vi "HTTPS Server Test.vi"() -> ()   [LabVIEW 2013]
uses:
  NI OpenSSL Socket/SSL_Lib/SSL-Lib/Library Paths.ctl
  NI OpenSSL Socket/SSL_Lib/SSL/SSL_Mode.ctl
  NI OpenSSL Socket/SSL_Lib/SSL-Lib/SSL-Lib.lvclass
  NI OpenSSL Socket/SSL_Lib/SSL-Context/SSL-Context.lvclass
  NI OpenSSL Socket/SSL_Lib/BIO/BIO.lvclass
  NI OpenSSL Socket/SSL_Lib/SSL/SSL.lvclass
panel:
  out "listener":i32
  out "accept":i32
  in  "String write":string="Hello!"
  out "String read":string
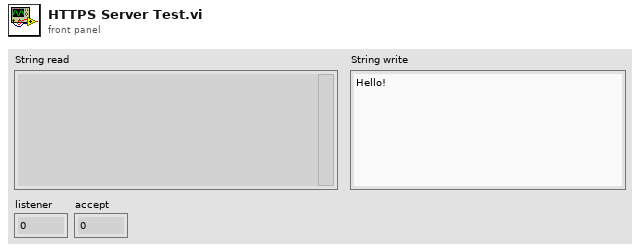
[diagram p1: front panel]
types:
  T1 = typedef "OpenSSL Socket.lvlib/SSL.lvclass/SSL_Mode.ctl" = i32
  T2 = typedef "OpenSSL Socket.lvlib/SSL-Lib.lvclass/Library Paths.ctl" = cluster{"SSL Library Path":path, "Crypto Library Path":path}
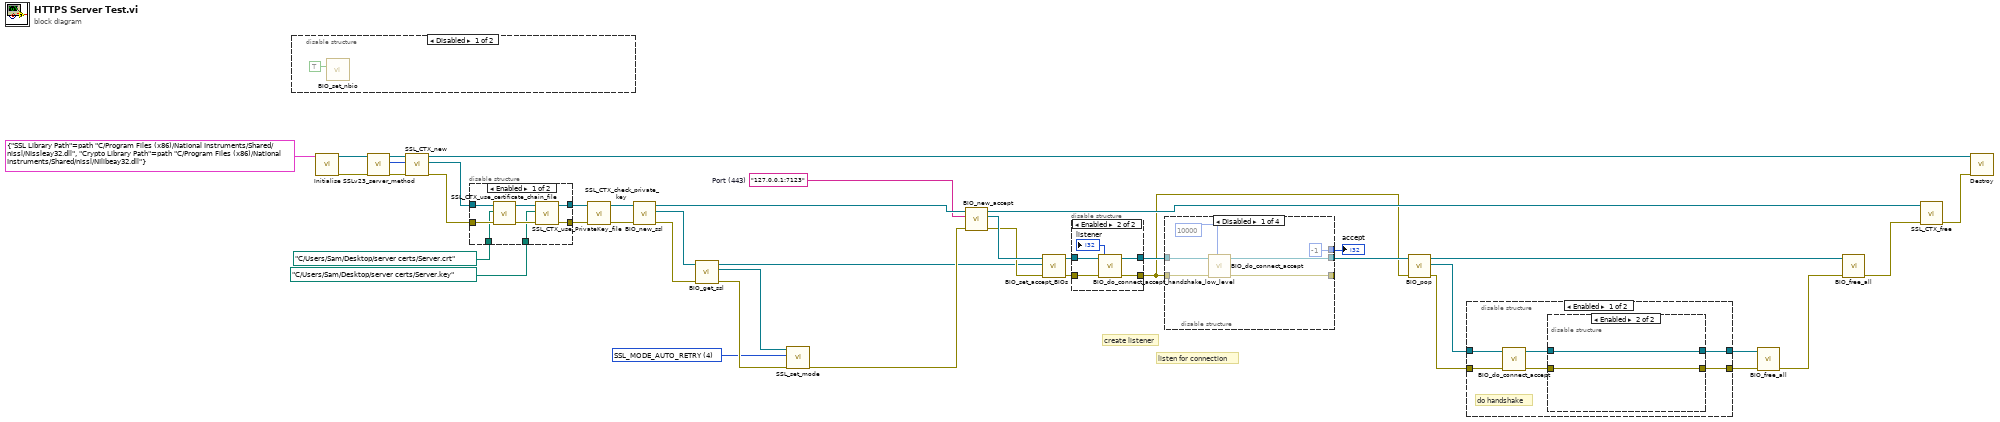
[diagram p0: block diagram]
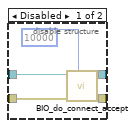
[diagram p2: hidden frame]
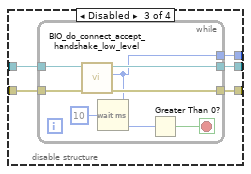
[diagram p4: hidden frame]
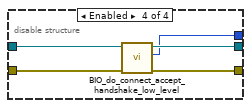
[diagram p5: hidden frame]
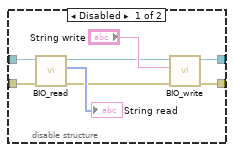
[diagram p6: hidden frame]
diagram:
  w15 = "127.0.0.1:7123"  # Port (443)
  w22 = T1 4 items=["None"=0, "SSL_MODE_ENABLE_PARTIAL_WRITE"=1, "SSL_MODE_ACCEPT_MOVING_WRITE_BUFFER"=2, "SSL_MODE_AUTO_RETRY"=4, "SSL_MODE_RELEASE_BUFFERS"=16, "SSL_MODE_SEND_FALLBACK_SCSV"=128] ("Mode")
  # "listen for connection"
  # "create listener"
  n1 = disable-structure shown="Disabled" {
    frame Disabled {
      n2 = call "BIO_set_nbio.vi"("Non-Blocking?"=TRUE) -> ()  [unwired: 9 in, 2 out]
    }
    frame Enabled {
    }
  }
  n3 = call "Initialise.vi"("Library Paths"=T2 {"SSL Library Path"=path "C:/Program Files (x86)/National Instruments/Shared/nissl/NIssleay32.dll", "Crypto Library Path"=path "C:/Program Files (x86)/National Instruments/Shared/nissl/NIlibeay32.dll"}) -> ("error out"=w37:errorcluster, "SSL-Lib out"=w41:refnum<class "SSL-Lib.lvclass">)  [unwired: 9 in]
  n4 = call "SSLv23_server_method.vi"("error in (no error)"=w37, "SSL-Lib in"=w41) -> ("error out"=w35:errorcluster, "*SSL_Method"=w40:u64, "SSL-Lib out"=w39:refnum<class "SSL-Lib.lvclass">)  [unwired: 7 in]
  n5 = call "SSL_CTX_new.vi"("error in (no error)"=w35, "*SSL_Method"=w40, "SSL-Lib in"=w39) -> ("error out"=w34:errorcluster, "SSL-Context out"=w33:refnum<class "SSL-Context.lvclass">, "SSL-Lib out"=w4:refnum<class "SSL-Lib.lvclass">)  [unwired: 6 in]
  n6 = disable-structure shown="Enabled" {
    disable-tunnel: w34 -> [w48 w51]
    disable-tunnel: w33 -> [w47 w52]
    disable-tunnel: [w46 w51] -> w32
    disable-tunnel: [w45 w52] -> w31
    disable-tunnel: path "C:/Users/Sam/Desktop/server certs/Server.crt" -> [w44 _]
    disable-tunnel: path "C:/Users/Sam/Desktop/server certs/Server.key" -> [w43 _]
    frame Enabled {
      n7 = call "SSL_CTX_use_certificate_chain_file.vi"("error in (no error)"=w48, "Certificate Chain File"=w44, "SSL-Context in"=w47) -> ("error out"=w50:errorcluster, "SSL-Context out"=w49:refnum<class "SSL-Context.lvclass">)  [unwired: 7 in]
      n8 = call "SSL_CTX_use_PrivateKey_file.vi"("error in (no error)"=w50, "PrivateKey File"=w43, "SSL-Context in"=w49) -> ("error out"=w46:errorcluster, "SSL-Context out"=w45:refnum<class "SSL-Context.lvclass">)  [unwired: 7 in]
    }
    frame Disabled {
    }
  }
  n9 = call "SSL_CTX_check_private_key.vi"("error in (no error)"=w32, "SSL-Context in"=w31) -> ("error out"=w30:errorcluster, "SSL-Context out"=w29:refnum<class "SSL-Context.lvclass">)  [unwired: 8 in]
  n10 = call "BIO_new_ssl.vi"("error in (no error)"=w30, "SSL-Context in"=w29) -> ("error out"=w25:errorcluster, "SSL BIO out"=w26:refnum<class "BIO.lvclass">, "SSL-Context out"=w19:refnum<class "SSL-Context.lvclass">)  [unwired: 7 in]
  n11 = call "BIO_get_ssl.vi"("error in (no error)"=w25, "BIO in"=w26) -> ("error out"=w23:errorcluster, "SSL out"=w24:refnum<class "SSL.lvclass">, "BIO out"=w2:refnum<class "BIO.lvclass">)  [unwired: 7 in]
  n12 = call "SSL_set_mode.vi"("error in (no error)"=w23, "Mode"=w22, "SSL in"=w24) -> ("error out"=w3:errorcluster)  [unwired: 7 in, 1 out]
  n13 = call "BIO_new_accept.vi"("error in (no error)"=w3, "Port (443)"=w15, "SSL-Context in"=w19) -> ("error out"=w16:errorcluster, "Accept BIO out"=w17:refnum<class "BIO.lvclass">, "SSL-Context out"=w18:refnum<class "SSL-Context.lvclass">)  [unwired: 6 in]
  n14 = call "BIO_set_accept_BIOs.vi"("error in (no error)"=w16, "SSL BIO"=w2, "Accept BIO in"=w17) -> ("error out"=w13:errorcluster, "Accept BIO out"=w14:refnum<class "BIO.lvclass">)  [unwired: 7 in]
  n15 = disable-structure shown="Enabled" {
    disable-tunnel: w14 -> [w56 w62]
    disable-tunnel: w13 -> [w55 w61]
    disable-tunnel: [w54 w59] -> w12
    disable-tunnel: [w53 w60] -> w5
    frame Disabled {
      n16 = call "BIO_do_connect_accept.vi"(7:u32 10000 ("Timeout (10000ms)"), "error in (no error)"=w55, "BIO in"=w56) -> ("error out"=w53:errorcluster, "BIO out"=w54:refnum<class "BIO.lvclass">)  [unwired: 7 in]
    }
    frame Enabled {
      n17 = call "BIO_do_connect_accept_handshake_low_level.vi"("error in (no error)"=w61, "BIO in"=w62) -> ("error out"=w60:errorcluster, "return type"=→"listener":i32, "BIO out"=w59:refnum<class "BIO.lvclass">)  [unwired: 7 in]
    }
  }
  n18 = disable-structure shown="Disabled" {
    disable-tunnel: w12 -> [w67 w70 w75 w87]
    disable-tunnel: w5 -> [w66 w69 w74 w86]
    disable-tunnel: [w65 w70 w73 w85] -> w10
    disable-tunnel: [w64 w69 w72 w84] -> _
    disable-tunnel: [-1 ("return type") _ w71 w83] -> w1
    frame Disabled {
      n19 = call "BIO_do_connect_accept.vi"(7:u32 10000 ("Timeout (10000ms)"), "error in (no error)"=w66, "BIO in"=w67) -> ("error out"=w64:errorcluster, "BIO out"=w65:refnum<class "BIO.lvclass">)  [unwired: 7 in]
    }
    frame Disabled {
    }
    frame Disabled {
      n20 = while {
        tunnel: w75 -> [w82]
        tunnel: w74 -> [w81]
        tunnel: [w80] -> w73
        tunnel: [w79] -> w72
        tunnel: [w76] -> w71
        stop <- w78 stop-if-true
        n21 = call "BIO_do_connect_accept_handshake_low_level.vi"("error in (no error)"=w81, "BIO in"=w82) -> ("error out"=w79:errorcluster, "return type"=w76:i32, "BIO out"=w80:refnum<class "BIO.lvclass">)  [unwired: 7 in]
        n22 = Wait (ms)(milliseconds to wait=u32 10) -> ()  [unwired: 1 out]
        n23 = Greater Than 0?(x=w76) -> (x > 0?=w78:bool)
      }
    }
    frame Enabled {
      n24 = call "BIO_do_connect_accept_handshake_low_level.vi"("error in (no error)"=w86, "BIO in"=w87) -> ("error out"=w84:errorcluster, "return type"=w83:i32, "BIO out"=w85:refnum<class "BIO.lvclass">)  [unwired: 7 in]
    }
  }
  "accept" <- w1
  n25 = call "BIO_pop.vi"("error in (no error)"=w5, "BIO in"=w10) -> ("error out"=w7:errorcluster, "Popped BIO"=w8:refnum<class "BIO.lvclass">, "BIO out"=w9:refnum<class "BIO.lvclass">)  [unwired: 7 in]
  n26 = disable-structure shown="Enabled" {
    disable-tunnel: [w93 w104] -> w21
    disable-tunnel: [w92 w105] -> w20
    disable-tunnel: w8 -> [w91 w105]
    disable-tunnel: w7 -> [w90 w104]
    frame Enabled {
      # "do handshake"
      n27 = call "BIO_do_connect_accept.vi"("error in (no error)"=w90, "BIO in"=w91) -> ("error out"=w89:errorcluster, "BIO out"=w88:refnum<class "BIO.lvclass">)  [unwired: 8 in]
      n28 = disable-structure shown="Enabled" {
        disable-tunnel: [w99 w103] -> w93
        disable-tunnel: [w98 w102] -> w92
        disable-tunnel: w89 -> [w95 w103]
        disable-tunnel: w88 -> [w94 w102]
        frame Disabled {
          n29 = call "BIO_read.vi"("error in (no error)"=w95, "BIO in"=w94) -> ("error out"=w96:errorcluster, "Bytes read"=→"String read":u8[], "BIO out"=w97:refnum<class "BIO.lvclass">)  [unwired: 7 in]
          n30 = call "BIO_write.vi"("error in (no error)"=w96, "Bytes to write"="String write", "BIO in"=w97) -> ("error out"=w99:errorcluster, "BIO out"=w98:refnum<class "BIO.lvclass">)  [unwired: 6 in, 1 out]
        }
        frame Enabled {
        }
      }
    }
    frame Disabled {
    }
  }
  n31 = call "BIO_free_all.vi"("error in (no error)"=w21, "BIO in"=w20) -> ("error out"=w6:errorcluster)  [unwired: 9 in]
  n32 = call "BIO_free_all.vi"("error in (no error)"=w6, "BIO in"=w9) -> ("error out"=w11:errorcluster)  [unwired: 9 in]
  n33 = call "SSL_CTX_free.vi"("error in (no error)"=w11, "SSL-Context in"=w18) -> ("error out"=w36:errorcluster)  [unwired: 9 in]
  n34 = call "Destroy.vi"("error in (no error)"=w36, "SSL-Lib in"=w4) -> ()  [unwired: 9 in, 1 out]
